vi "Purge.vi"(8 "error in (no error)":errorcluster) -> ()   [LabVIEW 2016]
uses:
  <vilib>/DAQmx/write.llb/DAQmx Write (Digital 1D Wfm NChan NSamp).vi
  <vilib>/DAQmx/create/channels.llb/DAQmx Create Channel (DO-Digital Output).vi
  <vilib>/DAQmx/configure/timing.llb/DAQmx Timing (Sample Clock).vi
  <resource>/objmgr/daqmx.rc
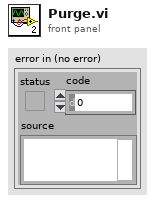
[diagram p1: front panel]
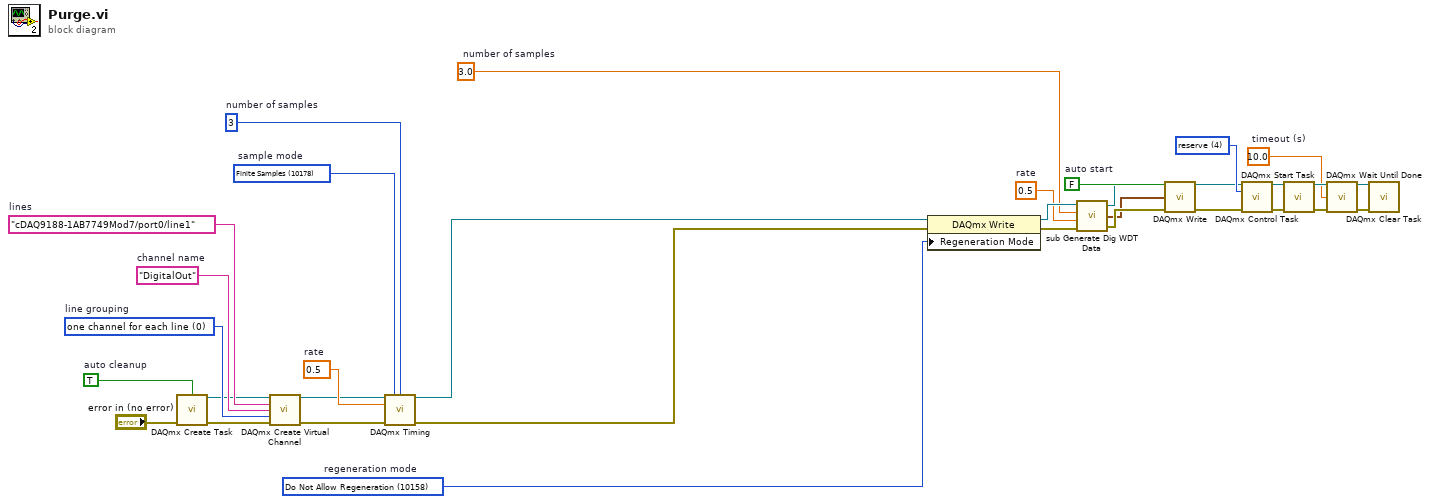
[diagram p0: block diagram]
diagram:
  w33 = 4 items=["verify"=2, "reserve"=4, "commit"=3, "unreserve"=5, "abort"=6] ("action")
  w26 = 10158 items=["Allow Regeneration"=10097, "Do Not Allow Regeneration"=10158]  # regeneration mode
  w24 = 10178 items=["Finite Samples"=10178, "Continuous Samples"=10123, "Hardware Timed Single Point"=12522]  # sample mode
  w23 = 3  # number of samples
  w22 = 0.5  # rate
  w17 = 0 items=["one channel for each line", "one channel for all lines"]  # line grouping
  w18 = "DigitalOut"  # channel name
  w16 = "cDAQ9188-1AB7749Mod7/port0/line1"  # lines
  w14 = TRUE  # auto cleanup
  w1 = 10.0  # timeout (s)
  w7 = 0.5  # rate
  w8 = 3.0  # number of samples
  w11 = FALSE  # auto start
  n1 = call <vilib>:"DAQmx Create Task.vi"("auto cleanup"=w14, "error in"="error in (no error)") -> ("task out"=w15:refnum<k21>, "error out"=w13:errorcluster)  [unwired: 12 in]
  n2 = call-poly <vilib>:"DAQmx Create Virtual Channel.vi"("task in"=w15, "lines"=w16, "name to assign"=w18, "line grouping"=w17, "error in"=w13) -> ("task out"=w21:refnum<k21>, "error out"=w19:errorcluster)  [unwired: 9 in]
  n3 = call-poly <vilib>:"DAQmx Timing.vi"("task/channels in"=w21, "sample mode"=w24, "samples per channel"=w23, "rate"=w22, "error in"=w19) -> ("task out"=w25:refnum<k21>, "error out"=w20:errorcluster)  [unwired: 9 in]
  n4 = property class="DAQmx Write"(reference=w25, error in=w20, "Regeneration Mode"=w26) -> (reference out=w27:refnum<k21>, error out=w28:errorcluster)
  n5 = call <vilib>:"sub Generate Dig WDT Data.vi"("task in"=w27, "number of samples"=w8, "update rate"=w7, "error in"=w28) -> ("task out"=w9:refnum<k21>, "data"=w2:digitalwaveform[], "error out"=w10:errorcluster)  [unwired: 1 in]
  n6 = call-poly <vilib>:"DAQmx Write.vi"("task/channels in"=w9, "auto start"=w11, "data"=w2, "error in"=w10) -> ("task out"=w29:refnum<k21>, "error out"=w31:errorcluster)  [unwired: 9 in, 1 out]
  n7 = call <vilib>:"DAQmx Control Task.vi"("task/channels in"=w29, "action"=w33, "error in"=w31) -> ("task out"=w30:refnum<k21>, "error out"=w32:errorcluster)  [unwired: 11 in]
  n8 = call <vilib>:"DAQmx Start Task.vi"("task/channels in"=w30, "error in"=w32) -> ("task out"=w6:refnum<k21>, "error out"=w5:errorcluster)  [unwired: 12 in]
  n9 = call <vilib>:"DAQmx Wait Until Done.vi"("task/channels in"=w6, "timeout (sec)"=w1, "error in"=w5) -> ("task out"=w3:refnum<k21>, "error out"=w4:errorcluster)  [unwired: 11 in]
  n10 = call <vilib>:"DAQmx Clear Task.vi"("task in"=w3, "error in"=w4) -> ()  [unwired: 13 in, 1 out]
